vi "globalSetUp.vi"(8 "error in (no error)":errorcluster, 11 "testcase-CSMGlobalLog in":refnum<class "testcase-CSMGlobalLog.lvclass">) -> (0 "error out":errorcluster, 3 "testcase-CSMGlobalLog out":refnum<class "testcase-CSMGlobalLog.lvclass">)   [LabVIEW 2017, in "testcase-CSMGlobalLog.lvclass"]
uses:
  testcase-CSMGlobalLog.lvclass
  <vilib>/addons/_JKI Toolkits/VI Tester/TestCase.llb/TestCase.lvclass
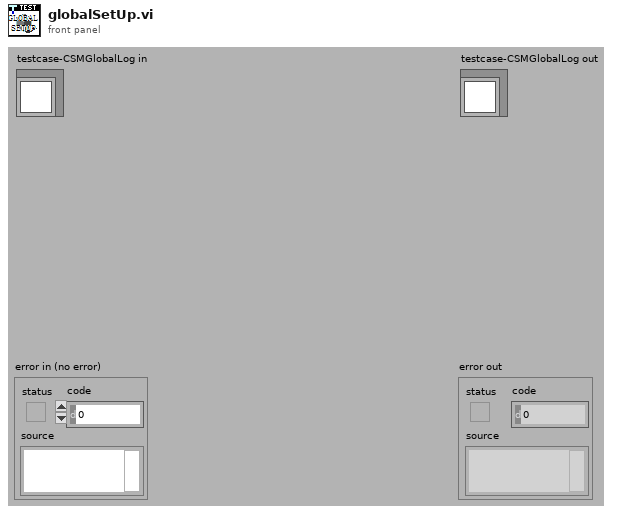
[diagram p1: front panel]
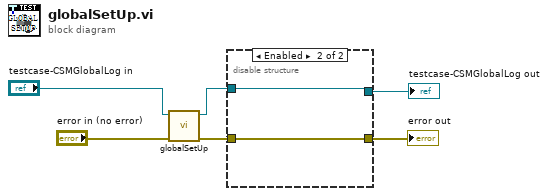
[diagram p0: block diagram]
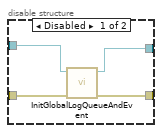
[diagram p2: hidden frame]
diagram:
  n1 = call-parent "globalSetUp.vi"("error in (no error)"="error in (no error)", "TestCase in"="testcase-CSMGlobalLog in") -> ("error out"=w3:errorcluster, "TestCase out"=w1:refnum<class "testcase-CSMGlobalLog.lvclass">)  [unwired: 8 in]
  n2 = disable-structure shown="Enabled" {
    disable-tunnel: w3 -> [w10 w11]
    disable-tunnel: [w9 w11] -> w6
    disable-tunnel: w1 -> [w8 w12]
    disable-tunnel: [w7 w12] -> w5
    frame Disabled {
      n3 = call "InitGlobalLogQueueAndEvent.vi"("error in (no error)"=w10, "TestCase in"=w8) -> ("error out"=w9:errorcluster, "TestCase out"=w7:refnum<class "testcase-CSMGlobalLog.lvclass">)  [unwired: 6 in, 2 out]
    }
    frame Enabled {
    }
  }
  "error out" <- w6
  "testcase-CSMGlobalLog out" <- w5
